vi "Transfer_SAT_Format.vi"(11 "SAT Outputs":T1={"D"=nan, "e"=nan, "h"=nan, "p"=nan, "s"=nan, "t"=nan, "q"=0.0, "Dl"=nan, "Dv"=nan, "x"=[nan, nan, 0.0, 0.0, 0.0, 0.0, 0.0, 0.0, 0.0, 0.0, 0.0, 0.0, 0.0, 0.0, 0.0, 0.0, 0.0, 0.0, 0.0, 0.0], "y"=[nan, nan, 0.0, 0.0, 0.0, 0.0, 0.0, 0.0, 0.0, 0.0, 0.0, 0.0, 0.0, 0.0, 0.0, 0.0, 0.0, 0.0, 0.0, 0.0], "nroot"=0, "k1"=0, "t1"=nan, "p1"=nan, "d1"=nan, "k2"=0, "t2"=nan, "p2"=nan, "d2"=nan, "k3"=0, "t3"=nan, "p3"=nan, "d3"=nan, "ierr"=0, "herr"="", "herr_length"=0}) -> (3 "Array out":dbl[](array[numeric]))   [LabVIEW 2021]
doc: "Converts output clusters from all SAT functions to an array of data."
uses:
  Ctl/SAT_Outputs.ctl
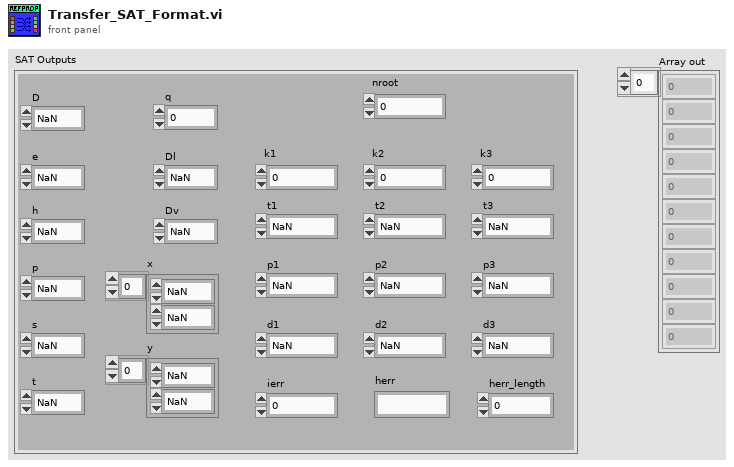
[diagram p1: front panel]
types:
  T1 = typedef "SAT_Outputs.ctl" = cluster{"D":dbl, "e":dbl, "h":dbl, "p":dbl, "s":dbl, "t":dbl, "q":dbl, "Dl":dbl, "Dv":dbl, "x":dbl[], "y":dbl[], "nroot":i32, "k1":i32, "t1":dbl, "p1":dbl, "d1":dbl, "k2":i32, "t2":dbl, "p2":dbl, "d2":dbl, "k3":i32, "t3":dbl, "p3":dbl, "d3":dbl, "ierr":i32, "herr":string, "herr_length":i32}
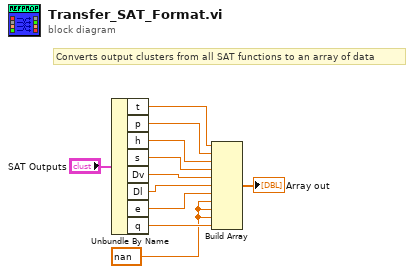
[diagram p0: block diagram]
diagram:
  w1 = nan ("w")
  # "Converts output clusters from all SAT functions to an array of data"
  n1 = Unbundle By Name("SAT Outputs") -> ("t"=w9:dbl, "p"=w8:dbl, "h"=w7:dbl, "s"=w6:dbl, "Dv"=w5:dbl, "Dl"=w4:dbl, "e"=w3:dbl, "q"=w2:dbl)
  n2 = Build Array(w9, w8, w7, w6, w5, w4, w3, w1, w1, w1, w2) -> (→"Array out":dbl[])
